vi "Flicker_Tablo_Doldur.vi"(10 "Table Reference in":refnum<vi>, 11 "Array In":dbl[][](array[numeric])) -> (1 "Test Result":bool, 2 "Table Values":string[][](array[string]), 3 "Array Out":dbl[][](array[numeric]))   [LabVIEW 2014]
panel:
  out "OlcumNo":u16
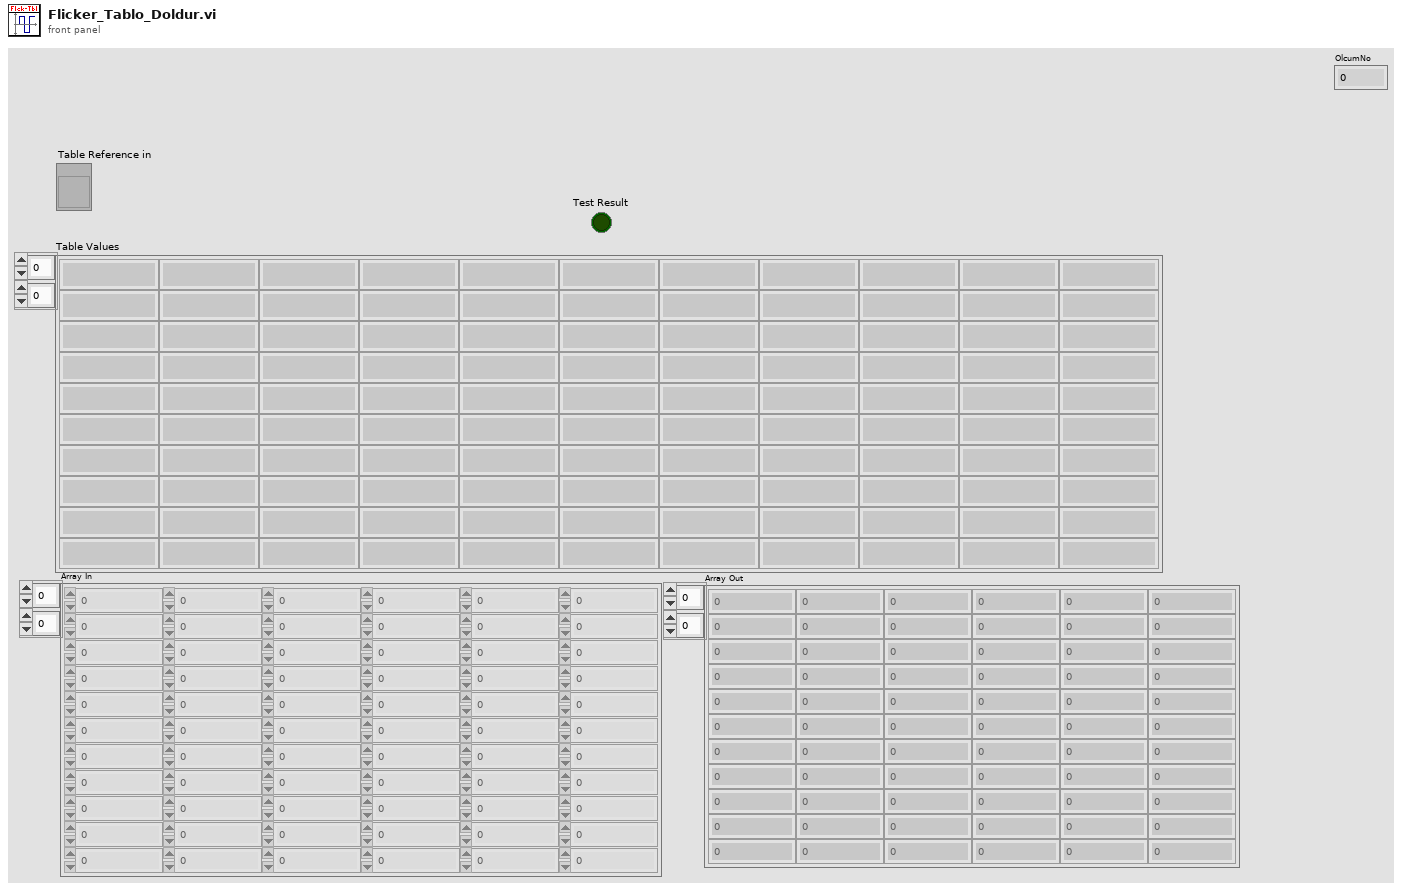
[diagram p1: front panel]
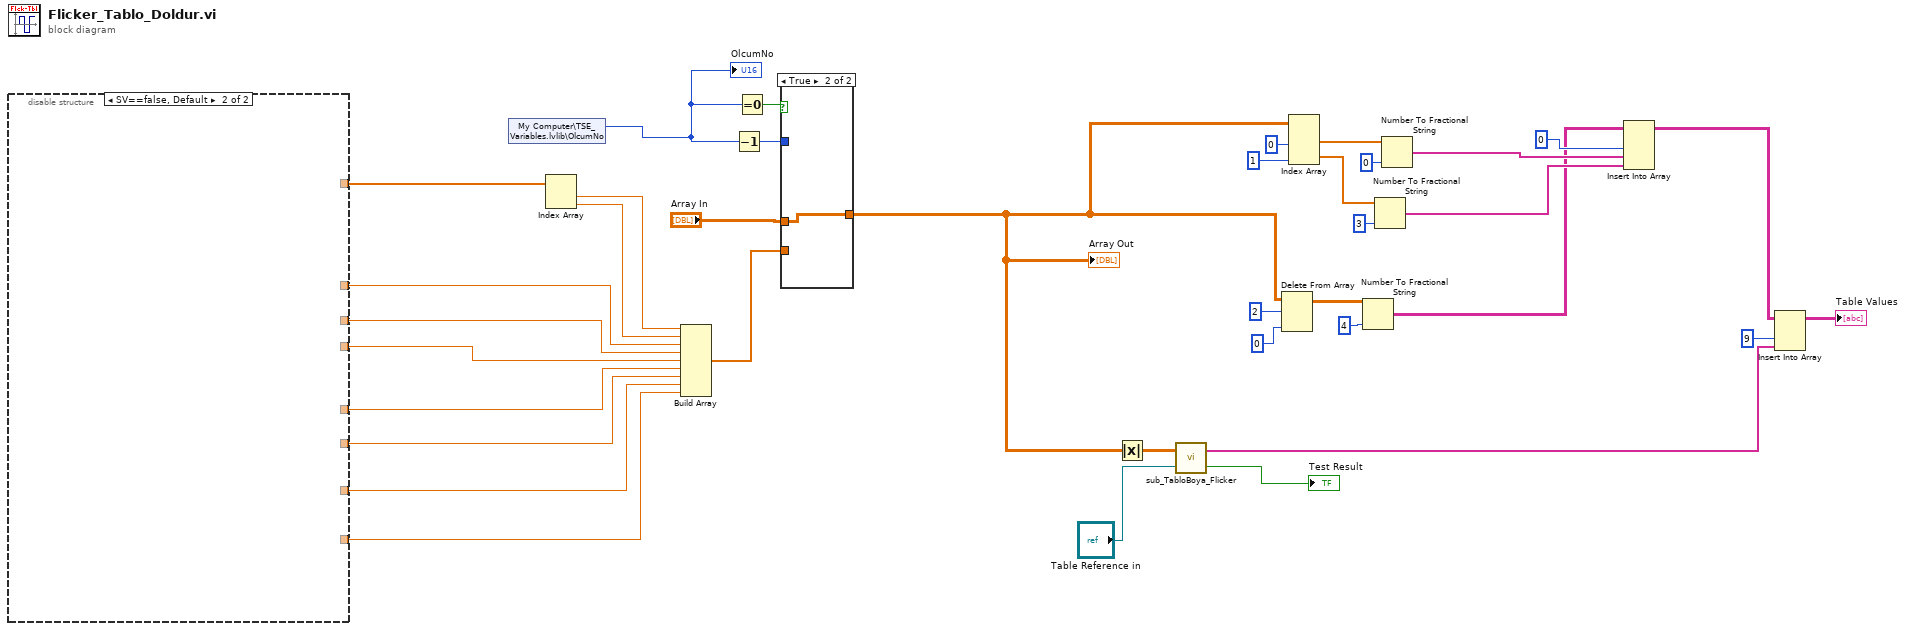
[diagram p0: block diagram]
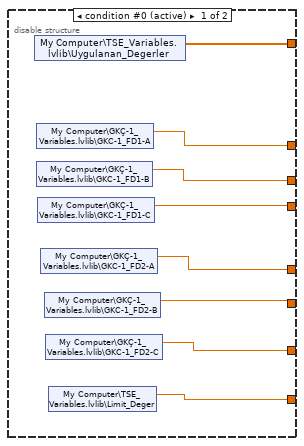
[diagram p2: hidden frame]
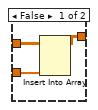
[diagram p3: hidden frame]
diagram:
  n1 = disable-structure shown="SV==false, Default" {
    disable-tunnel: [w45 _] -> w33
    disable-tunnel: [w44 _] -> w8
    disable-tunnel: [w43 _] -> w7
    disable-tunnel: [w42 _] -> w6
    disable-tunnel: [w41 _] -> w5
    disable-tunnel: [w40 _] -> w4
    disable-tunnel: [w39 _] -> w3
    disable-tunnel: [w38 _] -> w2
    frame condition #0 (active) {
      n2 = shared-variable "My Computer\\TSE_Variables.lvlib\\Uygulanan_Degerler"() -> (w45:dbl[])  [unwired: 1 in, 1 out]
      n3 = shared-variable "My Computer\\GKÇ-1_Variables.lvlib\\GKC-1_FD1-A"() -> (w44:dbl)  [unwired: 1 in, 1 out]
      n4 = shared-variable "My Computer\\GKÇ-1_Variables.lvlib\\GKC-1_FD1-B"() -> (w43:dbl)  [unwired: 1 in, 1 out]
      n5 = shared-variable "My Computer\\GKÇ-1_Variables.lvlib\\GKC-1_FD1-C"() -> (w42:dbl)  [unwired: 1 in, 1 out]
      n6 = shared-variable "My Computer\\GKÇ-1_Variables.lvlib\\GKC-1_FD2-A"() -> (w41:dbl)  [unwired: 1 in, 1 out]
      n7 = shared-variable "My Computer\\GKÇ-1_Variables.lvlib\\GKC-1_FD2-B"() -> (w40:dbl)  [unwired: 1 in, 1 out]
      n8 = shared-variable "My Computer\\GKÇ-1_Variables.lvlib\\GKC-1_FD2-C"() -> (w39:dbl)  [unwired: 1 in, 1 out]
      n9 = shared-variable "My Computer\\TSE_Variables.lvlib\\Limit_Deger"() -> (w38:dbl)  [unwired: 1 in, 1 out]
    }
    frame condition #1 {
    }
  }
  n10 = shared-variable "My Computer\\TSE_Variables.lvlib\\OlcumNo"() -> (w1:u16)  [unwired: 1 in, 1 out]
  "OlcumNo" <- w1
  n11 = Index Array(array=w33) -> (element #1=w32:dbl, element #2=w34:dbl)  [unwired: 2 in]
  n12 = Build Array(w32, w34, w8, w7, w6, w5, w4, w3, w2) -> (w28:dbl[])
  n13 = Decrement(x=w1) -> (x-1=w30:u16)
  n14 = Equal To 0?(x=w1) -> (x = 0?=w29:bool)
  n15 = case shown="True" w29 {
    tunnel: w28 -> [w47 _]
    tunnel: [w46 w49] -> w15
    tunnel: "Array In" -> [w48 w49]
    tunnel: w30 -> [_ _]
    frame False {
      n16 = Insert Into Array(array=w48, new element=w47) -> (w46:dbl[][])  [unwired: 2 in]
    }
    frame True {
    }
  }
  "Array Out" <- w15
  n17 = Absolute Value(x=w15) -> (abs(x)=w9:dbl[][])
  n18 = call "sub_TabloBoya_Flicker.vi"("Table in"="Table Reference in", "Tablo Degerleri"=w9) -> ("Test Result"=→"Test Result":bool, "RESULTS"=w36:string[])
  n19 = Delete From Array "Delete From Array"(array=w15, length=2, index (col)=0 ("disabled index (col)")) -> (array with subset deleted=w14:dbl[][])  [unwired: 1 in, 1 out]
  n20 = Index Array "Index Array"(array=w15, index (col) #1=0 ("disabled index (col)"), index (col) #2=1 ("index (col)")) -> (element #1=w18:dbl[], element #2=w19:dbl[])  [unwired: 2 in]
  n21 = Number To Fractional String(number=w14, precision (6)=i16 4) -> (F-format string=w13:string[][])  [unwired: 2 in]
  n22 = Number To Fractional String(number=w19, precision (6)=i16 3) -> (F-format string=w22:string[])  [unwired: 2 in]
  n23 = Number To Fractional String(number=w18, precision (6)=i16 0) -> (F-format string=w25:string[])  [unwired: 2 in]
  n24 = Insert Into Array(array=w13, index (col)=0 ("disabled index (col)"), new element #1=w25, new element #2=w22) -> (w12:string[][])  [unwired: 1 in]
  n25 = Insert Into Array(array=w12, index (col)=9 ("disabled index (col)"), new element=w36) -> (→"Table Values":string[][])  [unwired: 1 in]
